vi "FPGA open if close.vi"(8 "error in":errorcluster) -> (0 "error out":errorcluster, 2 "FPGA VI Reference Out":T1)   [LabVIEW 2019, in "my FPGA lib.lvlib"]
uses:
  my FPGA lib.lvlib
  FPPGA.ctl
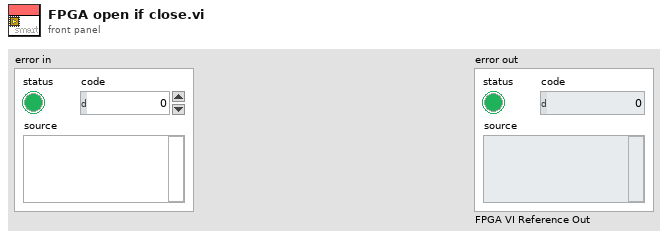
[diagram p1: front panel]
types:
  T1 = typedef "my FPGA lib.lvlib/FPPGA.ctl" = refnum<k20>
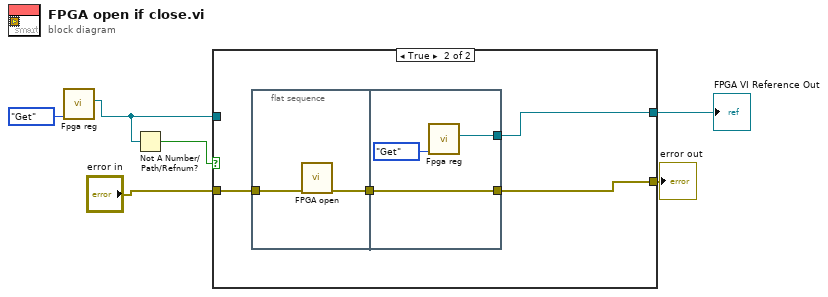
[diagram p0: block diagram]
diagram:
  n1 = call "Fpga reg.vi"("Mode"=enum16{"Get", "Set"}."Get") -> ("FPGA VI Reference Out"=w1:T1)  [unwired: 10 in]
  n2 = Not A Number/Path/Refnum?(number/path/refnum=w1) -> (NaN/Path/Refnum?=w5:bool)
  n3 = case shown="True" w5 {
    tunnel: "error in" -> [w7 w12]
    tunnel: [w7 w11] -> w3
    tunnel: [w8 w9] -> w2
    tunnel: w1 -> [w8 _]
    frame False {
    }
    frame True {
      n4 = flat-sequence {
        tunnel: w12 -> [w14]
        tunnel: [w13] -> w10
        tunnel: [w17] -> w11
        tunnel: w10 -> [w17]
        tunnel: [w15] -> w9
        frame #0 {
          n5 = call "FPGA open.vi"("error in"=w14) -> ("error out"=w13:errorcluster)  [unwired: 10 in]
        }
        frame #1 {
          n6 = call "Fpga reg.vi"("Mode"=enum16{"Get", "Set"}."Get") -> ("FPGA VI Reference Out"=w15:T1)  [unwired: 10 in]
        }
      }
    }
  }
  "error out" <- w3
  "FPGA VI Reference Out" <- w2
